vi "AutonVars.vi"() -> ()   [LabVIEW 2014]
panel:
  out "Autons":dbl[][](array[numeric])=[[-0.68, 2000.0, 3000.0, 0.0], [-0.68, 72.0, 2.0, 100.0]]
  # "Index\n\n0: OneBallAuton\n    0: Backward Speed\n    1: TimeDriveFoward (ms)\n    2: WaitTime (ms)\n\n1: TwoBallAuton\n    0: BackwardSpeed\n    1: TargetDistance (in) ToFire\n    2: WaitTime (s)\n    3: TargetDistance (in) ToReload"
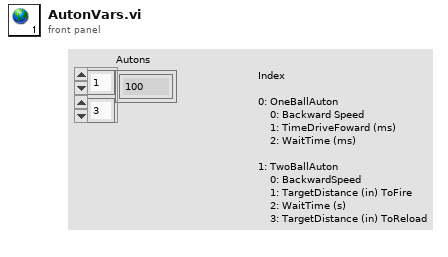
[diagram p1: front panel]
diagram:
